vi "Frame Rate ROI.vi"(2 "ROI":T1={"Horizontal Offset"=0, "Vertical Offset"=0, "Horizontal Width"=512, "Vertical Width"=512}, 3 "Exposure (ms)":dbl=0.1, 4 "Binning":u16(ring)=1 items=["1x1"=1, "2x2"=2, "4x4"=4]) -> (0 "Dropped Frames":i32=975, 1 "Frame Rate":dbl)   [LabVIEW 2013]
uses:
  <vilib>/Platform/TimedLoop/XDataNode/timing_clust.ctl
  <vilib>/Platform/TimedLoop/XDataNode/nitl_modes.ctl
  <vilib>/Platform/TimedLoop/XDataNode/wakeup.ctl
  <vilib>/platform/TimedLoop/XDataNode/XDataNode.xnode
  <vilib>/Platform/TimedLoop/XDataNode/XDNodeRunTimeDep.lvlib
panel:
  out "Elapsed Time":string="0 : 0 : 6.2"
  out "Total Frames":i32=1236
  out "Read Frames":i32=261
  out "Camera Info":string
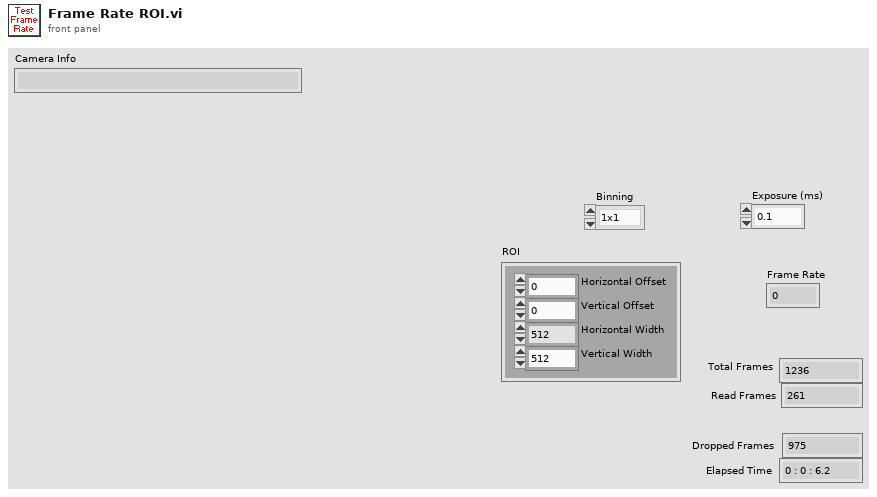
[diagram p1: front panel]
types:
  T1 = cluster{"Horizontal Offset":i32, "Vertical Offset":i32, "Horizontal Width":i32, "Vertical Width":i32}
  T2 = cluster{"height":u32, "width":u32, "datatype":u32}
  T3 = cluster{"Mode":u32, "Polarity":u32, "Period":dbl, "Delay":dbl}
  T4 = typedef "XDNodeRunTimeDep.lvlib/timing_clust.ctl" = cluster{"Expected End [f-1]":u64, "Actual End [f-1]":u64, "Finished Late? [f-1]":bool, "Expected End [i-1]":u64, "Actual End [i-1]":u64, "Finished Late? [i-1]":bool, "Expected Start [i]":u64, "Actual Start [i]":u64, "Expected Start [f]":u64, "Actual Start [f]":u64, "Source Name":string, "Structure Name":string, "Period":i64, "Deadline":i64, "Offset":i64, "Start":i64, "Priority":i32, "Timeout":i32, "Mode":T5, "Wakeup Reason":T6, "Error":errorcluster, "Source Type":string, "Secondary Source Type":string, "Global End Time":u64, "Global Start Time":u64, "Frame Duration":u64, "Iteration Duration":u64, "Assigned CPU":i32, "I/O Scan Engine Mode":u32}
  T5 = typedef "XDNodeRunTimeDep.lvlib/nitl_modes.ctl" = enum32{"No Change", "Process missed periods, maintain original phase", "Discard missed periods, maintain original phase", "Process missed periods, ignore original phase", "Discard missed periods, ignore original phase"}
  T6 = typedef "XDNodeRunTimeDep.lvlib/wakeup.ctl" = enum32{"Normal", "Aborted", "Asynchronous wakeup", "Timing source error", "Timed loop error", "Timeout"}
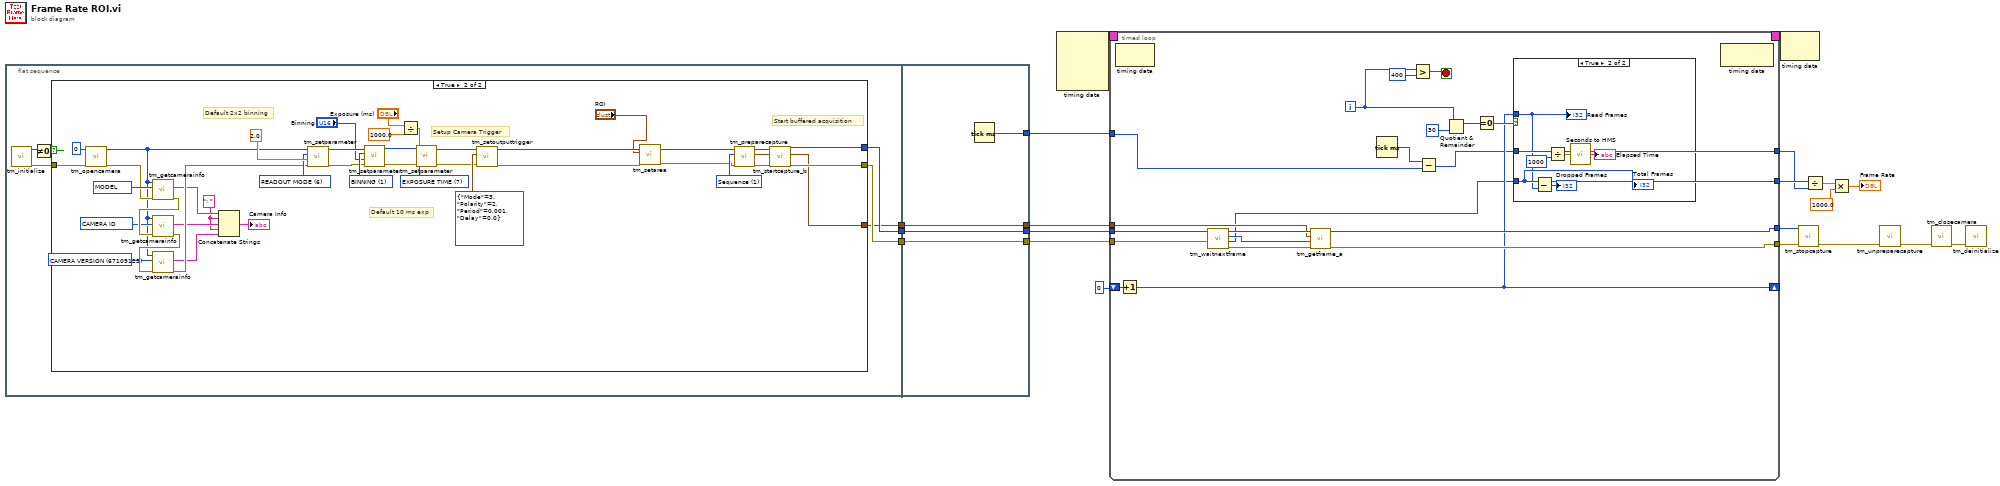
[diagram p0: block diagram]
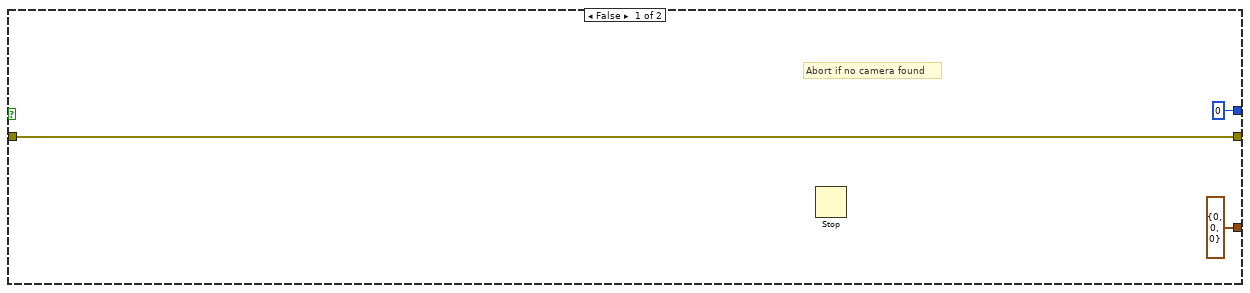
[diagram p2: hidden frame]
diagram:
  n1 = flat-sequence {
    tunnel: [w23] -> w9
    tunnel: [w22] -> w8
    tunnel: [w21] -> w7
    tunnel: [w72] -> w16
    tunnel: [w73] -> w17
    tunnel: [w74] -> w18
    tunnel: w9 -> [w74]
    tunnel: w8 -> [w73]
    tunnel: w7 -> [w72]
    tunnel: [w71] -> w6
    frame #0 {
      n2 = call <userlib>:"tm_initialize.vi"() -> ("error out"=w26:errorcluster, "Number Of Cameras"=w24:u32)  [unwired: 10 in]
      n3 = Not Equal To 0?(x=w24) -> (x != 0?=w25:bool)
      n4 = case shown="True" w25 {
        tunnel: w26 -> [w29 w70]
        tunnel: [u32 0 ("Handle out") w39] -> w23
        tunnel: [w29 w38] -> w22
        tunnel: [T2 {"height"=0, "width"=0, "datatype"=0} ("Buffer Info") w37] -> w21
        frame False {
          # "Abort if no camera found"
          n5 = Stop() -> ()  [unwired: 1 in]
        }
        frame True {
          w42 = "; " ("string")
          w58 = u32 6 items=["BINNING"=1, "BITS PER CHANNEL"=2, "ACTIVE VIEW INDEX"=3, "CCD MODE"=4, "SENSOR MODE"=5, "READOUT MODE"=6, "EXPOSURE TIME"=7, "CONTRAST GAIN"=8, "CONTRAST OFFSET"=9, "LIGHT MODE"=10, "SENSITIVITY"=11, "WHITE BALANCE"=12, "PHOTON IMAGING MODE"=13, "HIGH DYNAMIC RANGE MODE"=14, "TRIGGER SOURCE"=15, "TRIGGER ACTIVE"=16, "TRIGGER MODE"=17, "TRIGGER POLARITY"=18, "TRIGGER GLOBAL EXPOSURE"=19, "FIRST TRIGGER BEHAVIOR"=20, "TRIGGER TIMES"=21, "OUTPUT TRIGGER POLARITY"=22, "OUTPUT TRIGGER DELAY"=23, "OUTPUT TRIGGER PERIOD"=24, "TEMPERATURE"=25, "TEMPERATURE TARGET"=26, "SENSOR COOLER FAN"=27, "MECHANICAL SHUTTER"=28, "BACK FOCUS POSITION"=29, "FRAMEBUNDLE MODE"=30, "FRAMEBUNDLE NUMBER"=31, "LINEBUNDLE HEIGHT"=32, "TRIGGER CONNECTOR"=33, "IMAGE PIXEL TYPE"=34, "OUTPUT TRIGGER KIND"=35, "READOUT DIRECTION"=36, "CHANNEL SYNC"=37] ("Parameter")
          w60 = 1 items=["Snap", "Sequence"] ("Capture mode")
          w61 = u32 7 items=["BINNING"=1, "BITS PER CHANNEL"=2, "ACTIVE VIEW INDEX"=3, "CCD MODE"=4, "SENSOR MODE"=5, "READOUT MODE"=6, "EXPOSURE TIME"=7, "CONTRAST GAIN"=8, "CONTRAST OFFSET"=9, "LIGHT MODE"=10, "SENSITIVITY"=11, "WHITE BALANCE"=12, "PHOTON IMAGING MODE"=13, "HIGH DYNAMIC RANGE MODE"=14, "TRIGGER SOURCE"=15, "TRIGGER ACTIVE"=16, "TRIGGER MODE"=17, "TRIGGER POLARITY"=18, "TRIGGER GLOBAL EXPOSURE"=19, "FIRST TRIGGER BEHAVIOR"=20, "TRIGGER TIMES"=21, "OUTPUT TRIGGER POLARITY"=22, "OUTPUT TRIGGER DELAY"=23, "OUTPUT TRIGGER PERIOD"=24, "TEMPERATURE"=25, "TEMPERATURE TARGET"=26, "SENSOR COOLER FAN"=27, "MECHANICAL SHUTTER"=28, "BACK FOCUS POSITION"=29, "FRAMEBUNDLE MODE"=30, "FRAMEBUNDLE NUMBER"=31, "LINEBUNDLE HEIGHT"=32, "TRIGGER CONNECTOR"=33, "IMAGE PIXEL TYPE"=34, "OUTPUT TRIGGER KIND"=35, "READOUT DIRECTION"=36, "CHANNEL SYNC"=37] ("Parameter")
          w62 = u32 1 items=["BINNING"=1, "BITS PER CHANNEL"=2, "ACTIVE VIEW INDEX"=3, "CCD MODE"=4, "SENSOR MODE"=5, "READOUT MODE"=6, "EXPOSURE TIME"=7, "CONTRAST GAIN"=8, "CONTRAST OFFSET"=9, "LIGHT MODE"=10, "SENSITIVITY"=11, "WHITE BALANCE"=12, "PHOTON IMAGING MODE"=13, "HIGH DYNAMIC RANGE MODE"=14, "TRIGGER SOURCE"=15, "TRIGGER ACTIVE"=16, "TRIGGER MODE"=17, "TRIGGER POLARITY"=18, "TRIGGER GLOBAL EXPOSURE"=19, "FIRST TRIGGER BEHAVIOR"=20, "TRIGGER TIMES"=21, "OUTPUT TRIGGER POLARITY"=22, "OUTPUT TRIGGER DELAY"=23, "OUTPUT TRIGGER PERIOD"=24, "TEMPERATURE"=25, "TEMPERATURE TARGET"=26, "SENSOR COOLER FAN"=27, "MECHANICAL SHUTTER"=28, "BACK FOCUS POSITION"=29, "FRAMEBUNDLE MODE"=30, "FRAMEBUNDLE NUMBER"=31, "LINEBUNDLE HEIGHT"=32, "TRIGGER CONNECTOR"=33, "IMAGE PIXEL TYPE"=34, "OUTPUT TRIGGER KIND"=35, "READOUT DIRECTION"=36, "CHANNEL SYNC"=37] ("Parameter")
          w63 = u32 67109122 items=["BUS"=67109121, "CAMERA ID"=67109122, "VENDOR"=67109123, "MODEL"=67109124, "CAMERA VERSION"=67109125, "DRIVER VERSION"=67109126, "MODULE VERSIOIN"=67109127, "DCAMAPI VERSION"=67109128] ("Info ID")
          w65 = u32 67109125 items=["BUS"=67109121, "CAMERA"=67109122, "VENDOR"=67109123, "MODEL"=67109124, "CAMERA VERSION"=67109125, "DRIVER VERSION"=67109126, "MODULE VERSIOIN"=67109127, "DCAMAPI VERSION"=67109128] ("Info ID")
          w68 = u32 67109124 items=["BUS"=67109121, "CAMERA"=67109122, "VENDOR"=67109123, "MODEL"=67109124, "CAMERA VERSION"=67109125, "DRIVER VERSION"=67109126, "MODULE VERSIOIN"=67109127, "DCAMAPI VERSION"=67109128] ("Info ID")
          # "Start buffered acquisition"
          # "Setup Camera Trigger"
          # "Default 10 ms exp"
          # "Default 2x2 binning"
          n6 = call <userlib>:"tm_opencamera.vi"("error in (no error)"=w70, "Camera Index"=u32 0) -> ("error out"=w64:errorcluster, "Handle out"=w48:u32)  [unwired: 8 in]
          n7 = call <userlib>:"tm_getcamerainfo.vi"("error in (no error)"=w64, "Info ID"=w68, "Handle in"=w48) -> ("error out"=w67:errorcluster, "String"=w45:string)  [unwired: 6 in, 1 out]
          n8 = call <userlib>:"tm_getcamerainfo.vi"("error in (no error)"=w67, "Info ID"=w63, "Handle in"=w48) -> ("error out"=w66:errorcluster, "String"=w44:string)  [unwired: 6 in, 1 out]
          n9 = call <userlib>:"tm_getcamerainfo.vi"("error in (no error)"=w66, "Info ID"=w65, "Handle in"=w48) -> ("error out"=w47:errorcluster, "String"=w43:string)  [unwired: 6 in, 1 out]
          n10 = Concatenate Strings(w45, w42, w44, w42, w43) -> (→"Camera Info":string)
          n11 = call <userlib>:"tm_setparameter.vi"("error in (no error)"=w47, "Value in"=2.0, "Parameter"=w58, "Handle in"=w48) -> ("error out"=w49:errorcluster, "Handle out"=w50:u32)  [unwired: 6 in]
          n12 = call <userlib>:"tm_setparameter.vi"("error in (no error)"=w49, "Value in"="Binning", "Parameter"=w62, "Handle in"=w50) -> ("error out"=w56:errorcluster, "Handle out"=w57:u32)  [unwired: 6 in]
          n13 = Divide(x="Exposure (ms)", y=1000.0) -> (x/y=w40:dbl)
          n14 = call <userlib>:"tm_setparameter.vi"("error in (no error)"=w56, "Value in"=w40, "Parameter"=w61, "Handle in"=w57) -> ("error out"=w52:errorcluster, "Handle out"=w51:u32)  [unwired: 6 in]
          n15 = call <userlib>:"tm_setoutputtrigger.vi"("error in (no error)"=w52, "Parameters"=T3 {"Mode"=3, "Polarity"=2, "Period"=0.001, "Delay"=0.0}, "Handle in"=w51) -> ("error out"=w33:errorcluster, "Handle out"=w34:u32)  [unwired: 7 in]
          n16 = call <userlib>:"tm_setarea.vi"("error in (no error)"=w33, "Sub Region"="ROI", "Handle in"=w34) -> ("error out"=w32:errorcluster, "Handle out"=w31:u32)  [unwired: 7 in]
          n17 = call <userlib>:"tm_preparecapture.vi"("error in (no error)"=w32, "Capture mode"=w60, "Handle in"=w31) -> ("error out"=w54:errorcluster, "Buffer Info"=w37:T2, "Handle out"=w55:u32)  [unwired: 5 in, 1 out]
          n18 = call <userlib>:"tm_startcapture_b.vi"("error in (no error)"=w54, "Handle in"=w55) -> ("error out"=w38:errorcluster, "Handle out"=w39:u32)  [unwired: 8 in]
        }
      }
    }
    frame #1 {
      n19 = Tick Count (ms)() -> (millisecond timer value=w71:u32)
    }
  }
  n20 = node-c288() -> (w20:T4)  [unwired: 4 in]
  n21 = timed-loop {
    timing: w20 -> [_]
    timing-out: [_] -> w19
    tunnel: w18 -> [w91]
    tunnel: w17 -> [w90]
    tunnel: w16 -> [w89]
    tunnel: [w88] -> w12
    tunnel: [w87] -> w11
    shift-right: [w81] -> _
    shift-left: 0 -> [w82]
    tunnel: w6 -> [w80]
    tunnel: [w79] -> w4
    tunnel: [w78] -> w5
    i -> [w76]
    stop <- w77 stop-if-true
    n22 = node-c288() -> ()  [unwired: 1 in, 1 out]
    n23 = Increment(x=w82) -> (x+1=w81:i32)
    n24 = call <userlib>:"tm_waitnextframe.vi"("error in (no error)"=w90, "Handle in"=w91) -> ("error out"=w94:errorcluster, "Frame Count"=w78:i32, "Frame Index"=w92:i32, "Handle out"=w93:u32)  [unwired: 6 in]
    n25 = call <userlib>:"tm_getframe_a.vi"("error in (no error)"=w94, "Frame Index"=w92, "Buffer Info"=w89, "Handle in"=w93) -> ("error out"=w87:errorcluster, "Handle out"=w88:u32)  [unwired: 3 in, 3 out]
    n26 = Tick Count (ms)() -> (millisecond timer value=w86:u32)
    n27 = Greater?(x=w76, y=400) -> (0:w77:bool)
    n28 = Subtract(x=w86, y=w80) -> (x-y=w79:u32)
    n29 = Quotient & Remainder(x=w76, y=30) -> (x-y*floor(x/y)=w84:i32)  [unwired: 1 out]
    n30 = Equal To 0?(x=w84) -> (x = 0?=w83:bool)
    n31 = case shown="True" w83 {
      tunnel: w79 -> [_ w98]
      tunnel: w78 -> [_ w96]
      tunnel: w81 -> [_ w95]
      frame False {
      }
      frame True {
        n32 = Subtract(x=w96, y=w95) -> (x-y=→"Dropped Frames":i32)
        n33 = Divide(x=w98, y=u32 1000) -> (x/y=w100:dbl)
        n34 = call "Seconds to HMS.vi"("Time Elapsed in Seconds"=w100) -> ("Time Elapsed (H : M : S)"=→"Elapsed Time":string)
        "Total Frames" <- w96
        "Read Frames" <- w95
      }
    }
    n35 = node-c288() -> ()  [unwired: 1 in, 1 out]
  }
  n36 = node-c288(w19) -> ()  [unwired: 1 out]
  n37 = call <userlib>:"tm_stopcapture.vi"("error in (no error)"=w11, "Handle in"=w12) -> ("error out"=w14:errorcluster)  [unwired: 8 in, 1 out]
  n38 = Divide(x=w5, y=w4) -> (x/y=w3:dbl)
  n39 = Multiply(x=w3, y=1000.0) -> (x*y=→"Frame Rate":dbl)
  n40 = call <userlib>:"tm_unpreparecapture.vi"("error in (no error)"=w14) -> ("error out"=w13:errorcluster)  [unwired: 9 in, 1 out]
  n41 = call <userlib>:"tm_closecamera.vi"("error in (no error)"=w13) -> ("error out"=w15:errorcluster)  [unwired: 10 in]
  n42 = call <userlib>:"tm_deinitialize.vi"("error in (no error)"=w15) -> ()  [unwired: 10 in, 1 out]
